vi "Write I64 1.vi"(8 "error in (no error)":errorcluster, 10 "1":i64, 11 "CIFTemplateNode in":refnum<class "CIFTemplateNode.lvclass">) -> (0 "error out":errorcluster, 3 "CIFTemplateNode out":refnum<class "CIFTemplateNode.lvclass">)   [LabVIEW 2021, in "CIFTemplateNode.lvclass"]
uses:
  CIFTemplateNode.lvclass
  CIFTemplateNode.lvclass/CIFTemplateNode.ctl
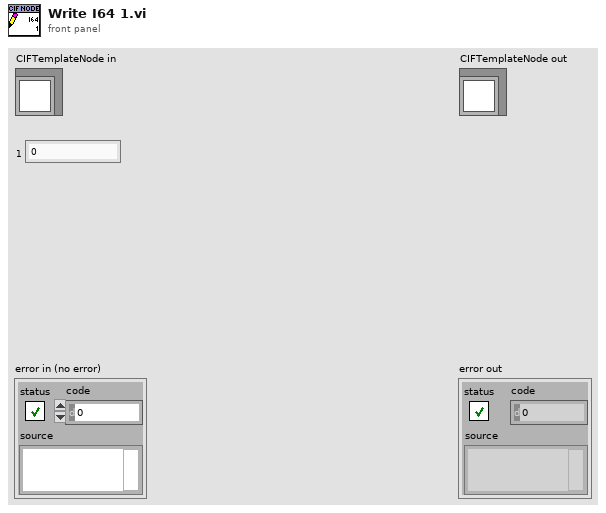
[diagram p1: front panel]
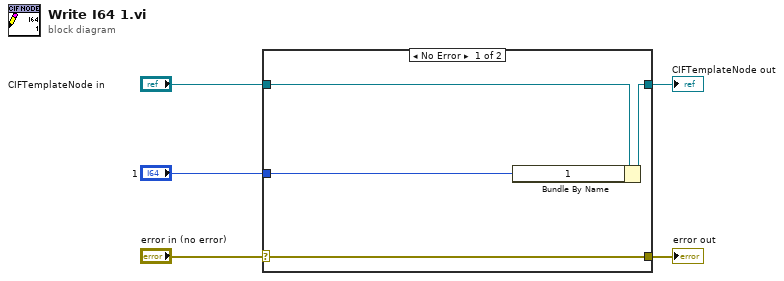
[diagram p0: block diagram]
diagram:
  n1 = case shown="No Error" "error in (no error)" {
    selector: "error in (no error)" -> [w9 w10]
    tunnel: [w9 w10] -> w4
    tunnel: [w7 w11] -> w2
    tunnel: "CIFTemplateNode in" -> [w8 w11]
    tunnel: "1" -> [w6 _]
    frame No Error {
      n2 = Bundle By Name(cluster=w8, "1"=w6) -> (w7:refnum<class "CIFTemplateNode.lvclass">)
    }
    frame Error {
    }
  }
  "error out" <- w4
  "CIFTemplateNode out" <- w2
